vi "CAN Initialize.vi"(6 "Interrupt":u16, 7 "IOPort":u32, 8 "error in (no error)":errorcluster, 9 "HwType":u8, 10 "Btr0Btr1":u16, 11 "Channel":u16) -> (0 "error out":errorcluster, 3 "TPCANStatus":u32)   [LabVIEW 2020, in "PCANBasic_eX.lvlib"]
doc: "TPCANStatus __stdcall CAN_Initialize(\n TPCANHandle Channel, \n TPCANBaudrate Btr0Btr1, \n TPCANType HwType _DEF_ARG,\n DWORD IOPort _DEF_ARG, \n WORD Interrupt _DEF_ARG);"
uses:
  PCANBasic_eX.lvlib
  PCANBasic.dll
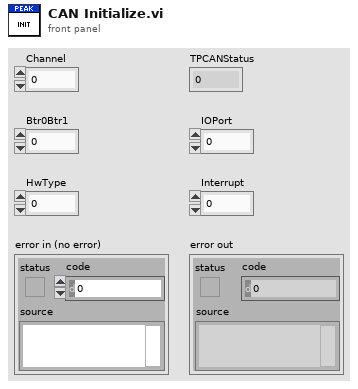
[diagram p1: front panel]
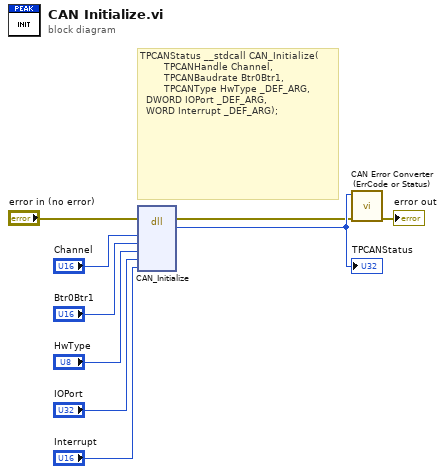
[diagram p0: block diagram]
diagram:
  # "TPCANStatus __stdcall CAN_Initialize(\n        TPCANHandle Channel, \n        TPCANBaudrate Btr0Btr1, \n        TPCANType HwType _DEF_ARG,\n\t\tDWORD IOPort _DEF_ARG, \n\t\tWORD Interrupt _DEF_ARG);"
  n1 = dll-call lib="PCANBasic.*" fn="CAN_Initialize"(error in="error in (no error)", "Channel"="Channel", "Btr0Btr1"="Btr0Btr1", "HwType"="HwType", "IOPort"="IOPort", "Interrupt"="Interrupt") -> (error out=w2:errorcluster, w9:u32)  [unwired: 7 in, 1 out]
  "TPCANStatus" <- w9
  n2 = call "CAN Error Converter (ErrCode or Status).vi"("error in (no error)"=w2, "error code"=w9) -> ("error out"=→"error out":errorcluster)  [unwired: 9 in]
